vi "LOG_GetLogPath.vi"(11 "logpath in":path) -> (3 "logpath out":path)   [LabVIEW 2016]
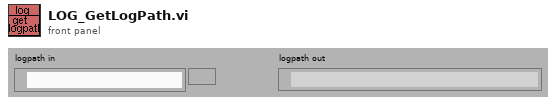
[diagram p1: front panel]
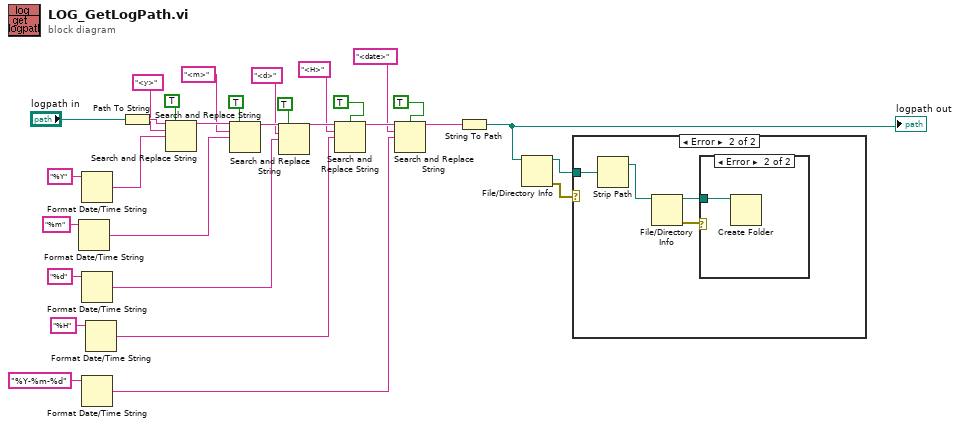
[diagram p0: block diagram]
diagram:
  n1 = Format Date/Time String(time format string (%c)="%m") -> (date/time string=w20:string)  [unwired: 2 out]
  n2 = Format Date/Time String(time format string (%c)="%Y") -> (date/time string=w26:string)  [unwired: 2 out]
  n3 = Format Date/Time String(time format string (%c)="%d") -> (date/time string=w17:string)  [unwired: 2 out]
  n4 = Format Date/Time String(time format string (%c)="%Y-%m-%d") -> (date/time string=w5:string)  [unwired: 2 out]
  n5 = Format Date/Time String(time format string (%c)="%H") -> (date/time string=w11:string)  [unwired: 2 out]
  n6 = Path To String(path="logpath in") -> (string=w30:string)
  n7 = Search and Replace String(replace all?=TRUE ("replace all? (F)"), input string=w30, search string="<y>", replace string=w26) -> (result string=w24:string)  [unwired: 1 in, 6 out]
  n8 = Search and Replace String(replace all?=TRUE ("replace all? (F)"), input string=w24, search string="<m>", replace string=w20) -> (result string=w18:string)  [unwired: 1 in, 6 out]
  n9 = Search and Replace String(replace all?=TRUE ("replace all? (F)"), input string=w18, search string="<d>", replace string=w17) -> (result string=w14:string)  [unwired: 1 in, 6 out]
  n10 = Search and Replace String(case sensitive?=TRUE ("replace all? (F)"), input string=w14, search string="<H>", replace string=w11) -> (result string=w9:string)  [unwired: 1 in, 6 out]
  n11 = Search and Replace String(case sensitive?=TRUE ("replace all? (F)"), input string=w9, search string="<date>", replace string=w5) -> (result string=w8:string)  [unwired: 1 in, 6 out]
  n12 = String To Path(string=w8) -> (path=w3:path)
  "logpath out" <- w3
  n13 = File/Directory Info(path=w3) -> (path out=w1:path, error out=w2:errorcluster)  [unwired: 1 in, 5 out]
  n14 = case shown="Error" w2 {
    tunnel: w1 -> [_ w34]
    frame No Error {
    }
    frame Error {
      n15 = Strip Path(path=w34) -> (stripped path=w33:path)  [unwired: 1 out]
      n16 = File/Directory Info(path=w33) -> (path out=w31:path, error out=w32:errorcluster)  [unwired: 1 in, 5 out]
      n17 = case shown="Error" w32 {
        tunnel: w31 -> [_ w35]
        frame No Error {
        }
        frame Error {
          n18 = Create Folder(path (use dialog)=w35) -> ()  [unwired: 1 in, 4 out]
        }
      }
    }
  }
